vi "Get Cache Path.vi"(8 "error in":errorcluster, 11 "Path Getter Mock in":refnum<class "Path Getter Mock.lvclass">) -> (0 "error out":errorcluster, 2 "Path":path)   [LabVIEW 2020, in "Path Getter Mock.lvclass"]
doc: "Returns a dummy Cache File for testing."
uses:
  Path Getter Mock.lvclass
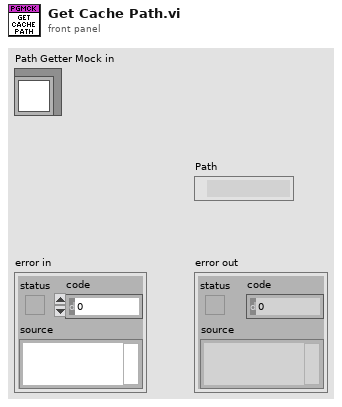
[diagram p1: front panel]
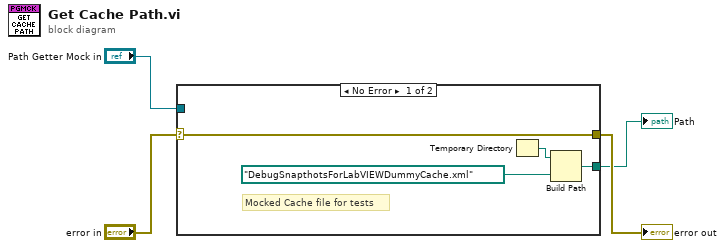
[diagram p0: block diagram]
diagram:
  n1 = case shown="No Error" "error in" {
    selector: "error in" -> [w8 w9]
    tunnel: [w5 _] -> w2
    tunnel: [w8 w9] -> w3
    tunnel: "Path Getter Mock in" -> [_ _]
    frame No Error {
      # "Mocked Cache file for tests"
      n2 = Temporary Directory() -> (w7:path)
      n3 = Build Path(base path=w7, name or relative path=path "DebugSnapthotsForLabVIEWDummyCache.xml") -> (appended path=w5:path)
    }
    frame Error {
    }
  }
  "error out" <- w3
  "Path" <- w2
